vi "Calculate Particle Scores Coral.vi"(6 "Limit":dbl=80.0 format="%#_13g", 10 "Sorted Data":dbl[][](array[numeric])) -> (3 "Scores":T1[](array[typedef]))   [LabVIEW 2025]
doc: "Calculate scores based on the particle measurements. Calculated scores are for aspect ratio, area to convex hull area, and moment of inertia. These scores range between 0 and 100 and can be used to categorize particles as targets and non-targets."
uses:
  Target Fields.ctl
  <vilib>/Analysis/baseanly.llb/Mean (DBL).vi
  <vilib>/Analysis/NI_AALBase.lvlib
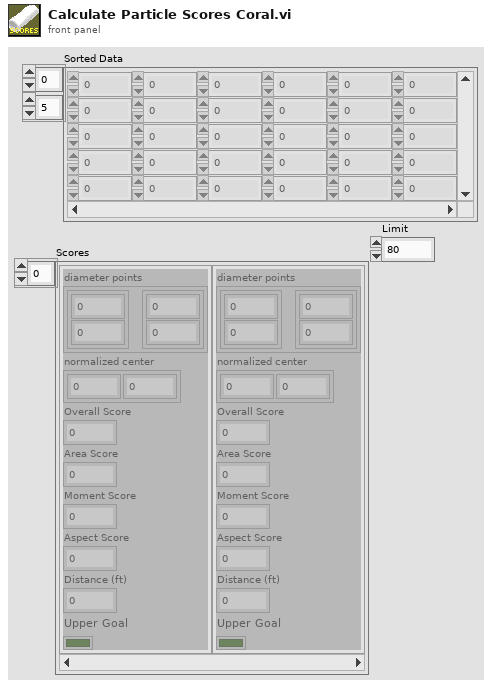
[diagram p1: front panel]
types:
  T1 = typedef "Target Fields.ctl" = cluster{"diameter points":cluster{"first point":cluster{"x":dbl, "y":dbl}, "projected point":cluster{"x":dbl, "y":dbl}}, "normalized center":cluster{"x":dbl, "y":dbl}, "Overall Score":dbl, "Area Score":dbl, "Moment Score":dbl, "Aspect Score":dbl, "Distance (ft)":dbl, "Upper Goal":bool}
  T2 = cluster{cluster{"Numeric":dbl, "Numeric":dbl}, cluster{"Numeric":dbl, "Numeric":dbl}}
  T3 = cluster{cluster{cluster{"Numeric":dbl, "Numeric":dbl}, cluster{"Numeric":dbl, "Numeric":dbl}}, "first point":cluster{"x":dbl, "y":dbl}, "mean":dbl, "Score":dbl, "Score":dbl, "Score":dbl, dbl, bool}
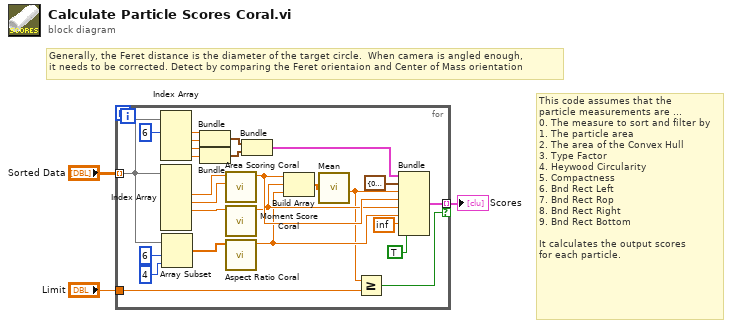
[diagram p0: block diagram]
diagram:
  # "Generally, the Feret distance is the diameter of the target circle.  When camera is angled enough,\nit needs to be corrected. Detect by comparing the Feret orientaion and Center of Mass orientation"
  # "This code assumes that the\nparticle measurements are ...\n0. The measure to sort and filter by\n1. The particle area\n2. The area of the Convex Hull\n3. Type Factor\n4. Heywood Circularity\n5. Compactness\n6. Bnd Rect Left\n7. Bnd Rect Rop\n8. Bnd Rect Right\n9. Bnd Rect Bottom\n\nIt calculates the output scores\nfor each particle."
  n1 = for {
    tunnel: "Sorted Data" -> [w5] mode=indexing
    tunnel: [w25] -> w2 mode=indexing if=w11
    tunnel: "Limit" -> [w16]
    n2 = Index Array(array=w5, index #1=6 ("index")) -> (element #1=w15:dbl, element #2=w14:dbl, element #3=w13:dbl, element #4=w12:dbl)  [unwired: 3 in]
    n3 = Index Array(array=w5) -> (element #2=w22:dbl, element #3=w17:dbl, element #4=w19:dbl)  [unwired: 6 in, 3 out]
    n4 = Array Subset(array=w5, index=6, length=4) -> (w4:dbl[])
    n5 = Bundle("Numeric"=w15, "Numeric"=w14) -> (w24:cluster{"Numeric":dbl, "Numeric":dbl})  [unwired: 1 in]
    n6 = Bundle("Numeric"=w13, "Numeric"=w12) -> (w23:cluster{"Numeric":dbl, "Numeric":dbl})  [unwired: 1 in]
    n7 = call "Area Scoring Coral.vi"("Convex Hull Area"=w17, "Area"=w22) -> ("Score"=w21:dbl)  [unwired: 9 in]
    n8 = call "Moment Score Coral.vi"("Moment Factor"=w19) -> ("Score"=w20:dbl)  [unwired: 10 in]
    n9 = call "Aspect Ratio Coral.vi"("Bounds"=w4) -> ("Score"=w18:dbl)  [unwired: 10 in]
    n10 = Bundle(w24, w23) -> (w28:T2)  [unwired: 1 in]
    n11 = Build Array(w21, w20, w18) -> (w9:dbl[])
    n12 = call-poly <vilib>:"Mean.vi"("X"=w9) -> ("mean"=w8:dbl)  [unwired: 1 out]
    n13 = Greater Or Equal?(x=w8, y=w16) -> (x >= y?=w11:bool)
    n14 = Bundle(w28, "first point"=cluster{"x":dbl, "y":dbl} {"x"=0.0, "y"=0.0}, "mean"=w8, "Score"=w21, "Score"=w20, "Score"=w18, inf, TRUE) -> (w25:T3)  [unwired: 1 in]
  }
  "Scores" <- w2
